vi "RightClickUpdate SliveAvg.vi"(8 "error in (no error)":errorcluster, 10 "Refs":T13, 11 "Loop data in":T2={"TitleCollapse"=refnum, "MouseDownState"=enum."Idle", "RightClickCache"={"Mod"={"Ctrl"=FALSE, "Shift"=FALSE}, "CoordsStart"={"Horizontal"=0, "Vertical"=0}, "CoordsEnd"={"Horizontal"=0, "Vertical"=0}, "PlotAreaBounds"={"Left"=10, "Top"=10, "Right"=0, "Bottom"=0}, "slice"=[]}, "ZoomCache"={"SuppressedPlots"=[], "LeftAxis"={"NeedsRevert?"=FALSE, "Scale Fit"=0, "Range"={"Minimum"=0.0, "Maximum"=0.0, "Increment"=0.0, "Minor Increment"=0.0, "Start"=0.0}}, "RightAxis"={"NeedsRevert?"=FALSE, "Scale Fit"=0, "Range"={"Minimum"=0.0, "Maximum"=0.0, "Increment"=0.0, "Minor Increment"=0.0, "Start"=0.0}}, "Mod"={"Shift"=FALSE}}, "UpdateTime"=0.0, "keyboard"=refnum, "visible?"=FALSE}) -> (0 "error out":errorcluster, 2 "cells":T1[][](array[typedef]), 3 "Loop data out":T2={"TitleCollapse"=refnum, "MouseDownState"=enum."Idle", "RightClickCache"={"Mod"={"Ctrl"=FALSE, "Shift"=FALSE}, "CoordsStart"={"Horizontal"=0, "Vertical"=0}, "CoordsEnd"={"Horizontal"=0, "Vertical"=0}, "PlotAreaBounds"={"Left"=10, "Top"=10, "Right"=0, "Bottom"=0}, "slice"=[]}, "ZoomCache"={"SuppressedPlots"=[], "LeftAxis"={"NeedsRevert?"=FALSE, "Scale Fit"=0, "Range"={"Minimum"=0.0, "Maximum"=0.0, "Increment"=0.0, "Minor Increment"=0.0, "Start"=0.0}}, "RightAxis"={"NeedsRevert?"=FALSE, "Scale Fit"=0, "Range"={"Minimum"=0.0, "Maximum"=0.0, "Increment"=0.0, "Minor Increment"=0.0, "Start"=0.0}}, "Mod"={"Shift"=FALSE}}, "UpdateTime"=0.0, "keyboard"=refnum, "visible?"=FALSE}, 4 "Row Headers":string[](array[string]), 6 "Column Headers":string[](array[string]))   [LabVIEW 2021, in "RocketPlot.lvlib"]
uses:
  RocketPlot.lvlib
  TypeDefs/Plot UI references.ctl
  Classes/RocketPlotHandle/RocketPlotHandle.lvclass
  <userlib>/bjustice/TipStripOOPanel/Classes/TipPanelHandle/TipPanelHandle.lvclass
  TypeDefs/Plot top row.ctl
  TypeDefs/plot while loop data.ctl
  CollapsePanel/CollapsePanel.lvclass
  TypeDefs/MouseDownState.ctl
  TypeDefs/RightClickCache.ctl
  TypeDefs/RightClickCache PlatMod.ctl
  <vilib>/Utility/miscctls.llb/LVPoint32TypeDef.ctl
  <vilib>/Utility/miscctls.llb/LVRectTypeDef.ctl
  TypeDefs/Slice average.ctl
  TypeDefs/ZoomCache.ctl
  TypeDefs/RangeCache.ctl
  <vilib>/Utility/miscctls.llb/LVRangeTypeDef.ctl
  TypeDefs/ZoomCache PlatMod.ctl
  Classes/TipTablePanel/cell cache.ctl
  Classes/TipTablePanel/TipTablePanel.lvclass
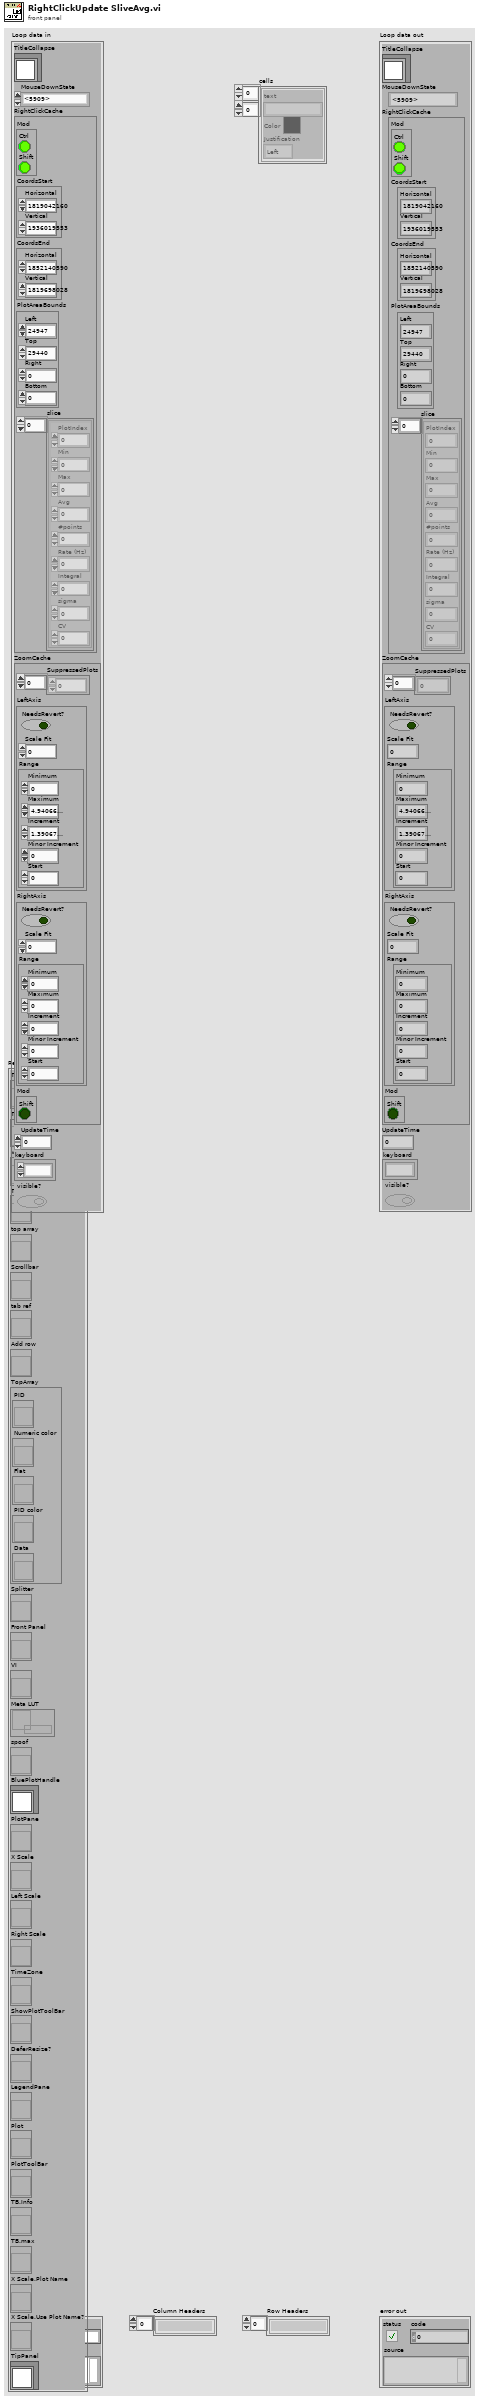
[diagram p1: front panel]
types:
  T1 = typedef "RocketPlot.lvlib/TipTablePanel.lvclass/cell cache.ctl" = cluster{"text":string, "Color":u32, "Justification":enum16{"Left", "Center", "Right"}}
  T2 = typedef "RocketPlot.lvlib/plot while loop data.ctl" = cluster{"TitleCollapse":refnum<class "CollapsePanel.lvclass">, "MouseDownState":T3, "RightClickCache":T4, "ZoomCache":T9, "UpdateTime":dbl, "keyboard":refnum<k1>, "visible?":bool}
  T3 = typedef "RocketPlot.lvlib/MouseDownState.ctl" = enum16{"Idle", "Pan", "Zoom", "Zoom-Post", "RightClick"}
  T4 = typedef "RocketPlot.lvlib/RightClickCache.ctl" = cluster{"Mod":T5, "CoordsStart":T6, "CoordsEnd":T6, "PlotAreaBounds":T7, "slice":T8[]}
  T5 = typedef "RocketPlot.lvlib/RightClickCache PlatMod.ctl" = cluster{"Ctrl":bool, "Shift":bool}
  T6 = typedef "LVPoint32TypeDef.ctl" = cluster{"Horizontal":i32, "Vertical":i32}
  T7 = typedef "LVRectTypeDef.ctl" = cluster{"Left":i16, "Top":i16, "Right":i16, "Bottom":i16}
  T8 = typedef "RocketPlot.lvlib/Slice average.ctl" = cluster{"PlotIndex":i32, "Min":dbl, "Max":dbl, "Avg":dbl, "#points":u32, "Rate (Hz)":dbl, "Integral":dbl, "sigma":dbl, "CV":dbl}
  T9 = typedef "RocketPlot.lvlib/ZoomCache.ctl" = cluster{"SuppressedPlots":i32[], "LeftAxis":T10, "RightAxis":T10, "Mod":T12}
  T10 = typedef "RocketPlot.lvlib/RangeCache.ctl" = cluster{"NeedsRevert?":bool, "Scale Fit":u8, "Range":T11}
  T11 = typedef "LVRangeTypeDef.ctl" = cluster{"Minimum":dbl, "Maximum":dbl, "Increment":dbl, "Minor Increment":dbl, "Start":dbl}
  T12 = typedef "RocketPlot.lvlib/ZoomCache PlatMod.ctl" = cluster{"Shift":bool}
  T13 = typedef "RocketPlot.lvlib/Plot UI references.ctl" = cluster{"Title":refnum<vi>, "Title?":refnum<vi>, "Visible sidebar?":refnum<vi>, "Time to Plot":refnum<vi>, "top array":refnum<vi>, "Scrollbar":refnum<vi>, "tab ref":refnum<vi>, "Add row":refnum<vi>, "TopArray":cluster{"PID":refnum<vi>, "Numeric color":refnum<vi>, "Flat":refnum<vi>, "PID color":refnum<vi>, "Data":refnum<vi>}, "Splitter":refnum<vi>, "Front Panel":refnum<vi>, "VI":refnum<vi>, "Meta LUT":refnum<data-value>, "spoof":refnum<vi>, "BluePlotHandle":refnum<class "RocketPlotHandle.lvclass">, "PlotPane":refnum<vi>, "X Scale":refnum<vi>, "Left Scale":refnum<vi>, "Right Scale":refnum<vi>, "TimeZone":refnum<vi>, "ShowPlotToolBar":refnum<vi>, "DeferResize?":refnum<vi>, "LegendPane":refnum<vi>, "Plot":refnum<vi>, "PlotToolBar":refnum<vi>, "TB.Info":refnum<vi>, "TB.max":refnum<vi>, "X Scale.Plot Name":refnum<vi>, "X Scale.Use Plot Name?":refnum<vi>, "TipPanel":refnum<class "TipPanelHandle.lvclass">}
  T14 = typedef "StokePlot.lvlib/Plot top row.ctl" = cluster{"PID":string, "index":i32, "PID color":u32, "right axis?":bool, "Flatline?":bool, "Numeric color":u32, "Data":string, "Flat":string}
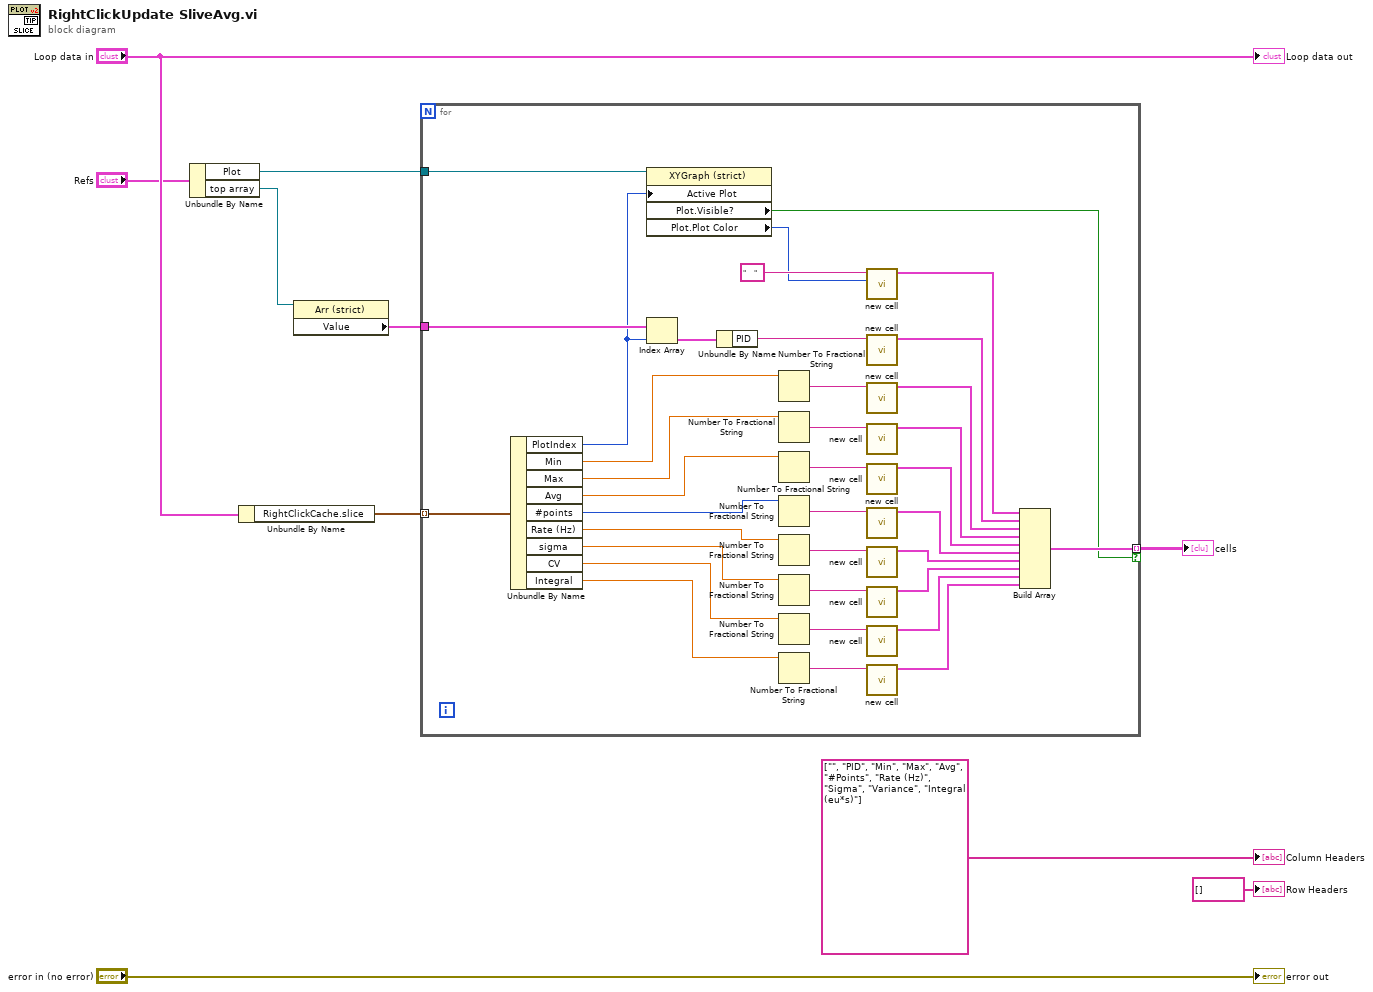
[diagram p0: block diagram]
diagram:
  n1 = Unbundle By Name("Refs") -> ("Plot"=w2:refnum<vi>, "top array"=w6:refnum<vi>)
  n2 = Unbundle By Name("Loop data in") -> ("RightClickCache.slice"=w10:T8[])
  n3 = property class="Arr (strict)"(reference=w6) -> ("Value"=w5:T14[])  [unwired: 1 in, 2 out]
  n4 = for {
    tunnel: w10 -> [w45] mode=indexing
    tunnel: [w46] -> w1 mode=indexing if=w32
    tunnel: w5 -> [w44]
    tunnel: w2 -> [w34]
    n5 = Unbundle By Name(w45) -> ("PlotIndex"=w33:i32, "Min"=w42:dbl, "Max"=w41:dbl, "Avg"=w35:dbl, "#points"=w40:u32, "Rate (Hz)"=w39:dbl, "sigma"=w38:dbl, "CV"=w37:dbl, "Integral"=w36:dbl)
    n6 = property class="XYGraph (strict)"(reference=w34, "Active Plot"=w33) -> ("Plot.Visible?"=w32:bool, "Plot.Plot Color"=w29:u32)  [unwired: 1 in, 2 out]
    n7 = Index Array(array=w44, index=w33) -> (element=w43:T14)
    n8 = Unbundle By Name(w43) -> ("PID"=w28:string)
    n9 = Number To Fractional String(number=w42) -> (F-format string=w26:string)  [unwired: 3 in]
    n10 = Number To Fractional String(number=w41) -> (F-format string=w24:string)  [unwired: 3 in]
    n11 = Number To Fractional String(number=w35) -> (F-format string=w22:string)  [unwired: 3 in]
    n12 = Number To Fractional String(number=w40) -> (F-format string=w20:string)  [unwired: 3 in]
    n13 = Number To Fractional String(number=w39) -> (F-format string=w18:string)  [unwired: 3 in]
    n14 = Number To Fractional String(number=w38) -> (F-format string=w16:string)  [unwired: 3 in]
    n15 = Number To Fractional String(number=w37) -> (F-format string=w14:string)  [unwired: 3 in]
    n16 = Number To Fractional String(number=w36) -> (F-format string=w12:string)  [unwired: 3 in]
    n17 = call "new cell.vi"("BG color"=w29, "String"="    ") -> ("cell"=w30:T1)  [unwired: 9 in]
    n18 = call "new cell.vi"("String"=w28) -> ("cell"=w27:T1)  [unwired: 10 in]
    n19 = call "new cell.vi"("String"=w26) -> ("cell"=w25:T1)  [unwired: 10 in]
    n20 = call "new cell.vi"("String"=w24) -> ("cell"=w23:T1)  [unwired: 10 in]
    n21 = call "new cell.vi"("String"=w22) -> ("cell"=w21:T1)  [unwired: 10 in]
    n22 = call "new cell.vi"("String"=w20) -> ("cell"=w19:T1)  [unwired: 10 in]
    n23 = call "new cell.vi"("String"=w18) -> ("cell"=w17:T1)  [unwired: 10 in]
    n24 = call "new cell.vi"("String"=w16) -> ("cell"=w15:T1)  [unwired: 10 in]
    n25 = call "new cell.vi"("String"=w14) -> ("cell"=w13:T1)  [unwired: 10 in]
    n26 = call "new cell.vi"("String"=w12) -> ("cell"=w11:T1)  [unwired: 10 in]
    n27 = Build Array(w30, w27, w25, w23, w21, w19, w17, w15, w13, w11) -> (w46:T1[])
  }
  "cells" <- w1
  "error out" <- "error in (no error)"
  "Loop data out" <- "Loop data in"
  "Row Headers" <- string[] [] ("Row Headers")
  "Column Headers" <- string[] ["", "PID", "Min", "Max", "Avg", "#Points", "Rate (Hz)", "Sigma", "Variance", "Integral (eu*s)"] ("Row Headers")
